vi "HelloWorldJP_copia.vi"() -> ()   [LabVIEW 2015]
panel:
  out "?":string
  out "appended array":bool[](array[boolean])
  out "number":u32
  out "length":i32
  in  "stop":bool
  in  "String in":string="Hola Mundo!"
  out "*(type *) &x":bool[](array[boolean])
  out "String out":string
  out "?":string
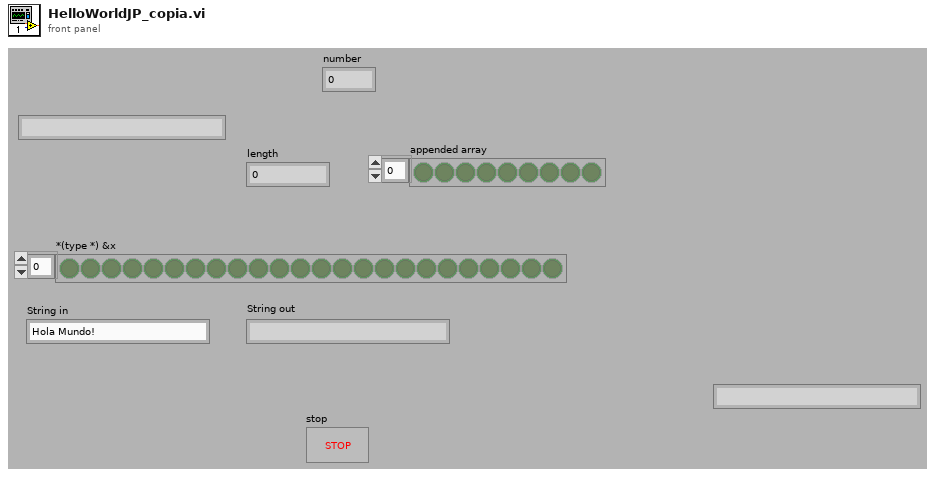
[diagram p1: front panel]
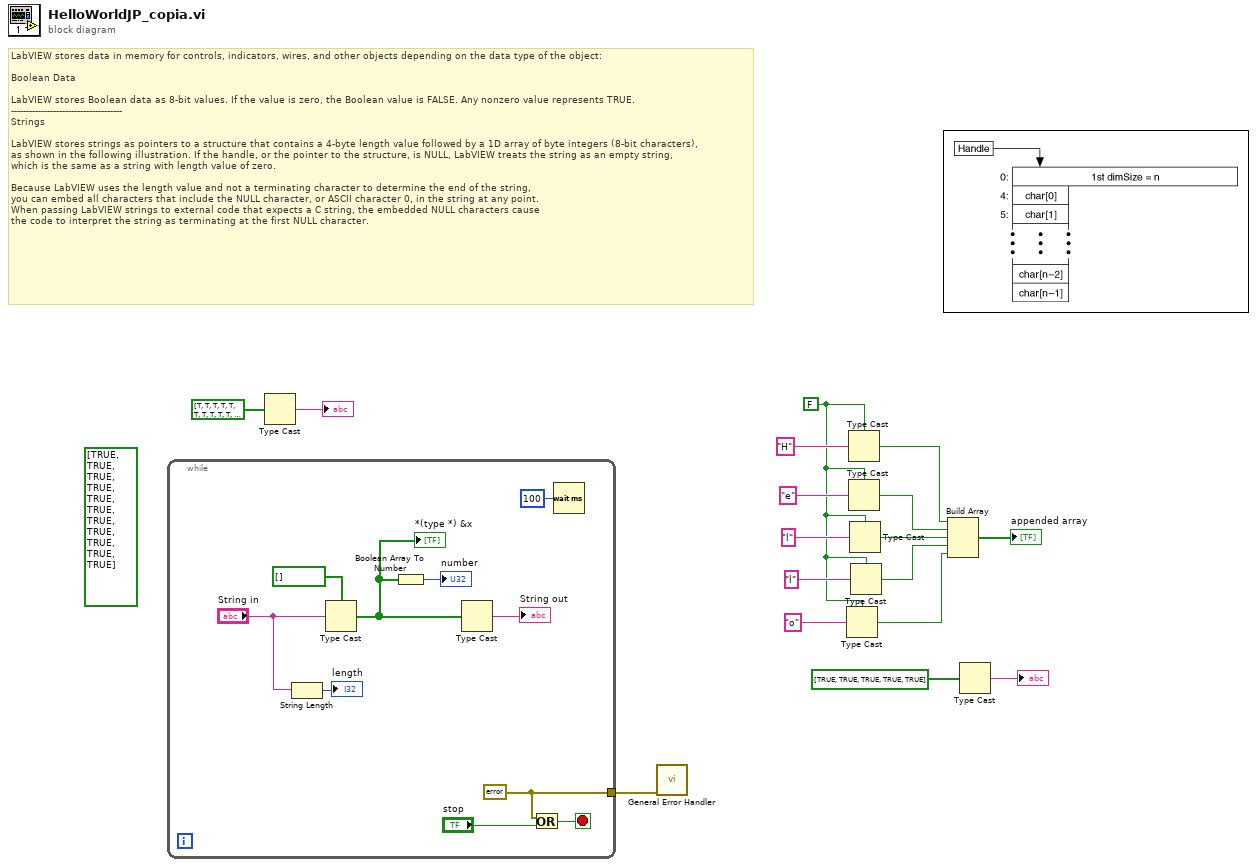
[diagram p0: block diagram]
diagram:
  w9 = FALSE
  (unwired) bool[] [TRUE, TRUE, TRUE, TRUE, TRUE, TRUE, TRUE, TRUE, TRUE, TRUE, TRUE] ("*(type *) &x")
  # "LabVIEW stores data in memory for controls, indicators, wires, and other objects depending on the data type of the object:\n\nBoolean Data\n\nLabVIEW stores Boolean data as 8-bit values. If the value is zero, the Boolean value is FALSE. Any nonzero value represents TRUE.\n-------------------------------------\nStrings\n\nLabVIEW stores strings as pointers to a structure that contains a 4-byte length value followed by a 1D array of byte integers (8-bit characters), \nas shown in the following illustration. If the handle, or the pointer to the structure, is NULL, LabVIEW treats the string as an empty string, \nwhich is the same as a string with length value of zero. \n\nBecause LabVIEW uses the length value and not a terminating character to determine the end of the string, \nyou can embed all characters that include the NULL character, or ASCII character 0, in the string at any point. \nWhen passing LabVIEW strings to external code that expects a C string, the embedded NULL characters cause \nthe code to interpret the string as terminating at the first NULL character."
  n1 = while {
    tunnel: [w18] -> w15
    stop <- w23 stop-if-true
    w18 = errorcluster {"status"=FALSE, "code"=0, "source"=""} ("error constant")
    n2 = String Length(string="String in") -> (length=→"length":i32)
    n3 = Type Cast(type=bool[] [], x="String in") -> (*(type *) &x=w20:bool[])
    "*(type *) &x" <- w20
    n4 = Boolean Array To Number(Boolean array=w20) -> (number=→"number":u32)
    n5 = Type Cast(x=w20) -> (*(type *) &x=→"String out":string)  [unwired: 1 in]
    n6 = Or(x=w18, y="stop") -> (x .or. y?=w23:bool)
    n7 = Wait (ms)(milliseconds to wait=u32 100) -> ()  [unwired: 1 out]
  }
  n8 = Type Cast(x=bool[] [TRUE, TRUE, TRUE, TRUE, TRUE, TRUE, TRUE, TRUE, TRUE, TRUE, TRUE, TRUE] ("*(type *) &x")) -> (*(type *) &x=→"?":string)  [unwired: 1 in]
  n9 = call <vilib>:"General Error Handler.vi"("error in (no error)"=w15) -> ()  [unwired: 10 in, 5 out]
  n10 = Type Cast(type=w9, x="o") -> (*(type *) &x=w4:bool)
  n11 = Type Cast(type=w9, x="H") -> (*(type *) &x=w8:bool)
  n12 = Type Cast(type=w9, x="e") -> (*(type *) &x=w7:bool)
  n13 = Type Cast(type=w9, x="l") -> (*(type *) &x=w6:bool)
  n14 = Type Cast(type=w9, x="l") -> (*(type *) &x=w5:bool)
  n15 = Build Array(w8, w7, w6, w5, w4) -> (→"appended array":bool[])
  n16 = Type Cast(x=bool[] [TRUE, TRUE, TRUE, TRUE, TRUE] ("appended array")) -> (*(type *) &x=→"?":string)  [unwired: 1 in]
